vi "GetProperties.vi"(8 "error in":errorcluster, 11 "Path in":refnum<class "Path.lvclass">) -> (0 "error out":errorcluster, 3 "Path out":refnum<class "Path.lvclass">)   [LabVIEW 2014, in "Path.lvclass"]
uses:
  Path.lvclass
  Path.lvclass/Path.ctl
  Control/Control.lvclass
  Text/Text.lvclass
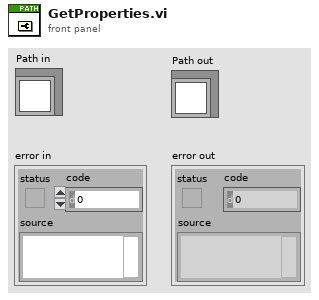
[diagram p1: front panel]
types:
  T1 = typedef "LVRectTypeDef.ctl" = cluster{"Left":i16, "Top":i16, "Right":i16, "Bottom":i16}
  T2 = typedef "LVBrowseOptionsTypeDef.ctl" = cluster{"Prompt":string, "Match Pattern":string, "select mode":enum32{"existing file", "new file", "new or existing file", "existing dir", "new dir", "new or existing dir", "existing file (use LLBs)", "new file (use LLBs)", "new or existing file (use LLBs)", "new or existing file or directory (use LLBs)", "existing dir (use LLBs)", "new dir (use LLBs)", "new or existing dir (use LLBs)", "existing file or dir", "new file or dir", "new or existing file or dir", "existing file or dir (use LLBs)", "new file or dir (use LLBs)"}, "Start Path":path, "Pattern Label":string, "Button Text":string}
  T3 = typedef "LVBoundsTypeDef.ctl" = cluster{"Width":u32, "Height":u32}
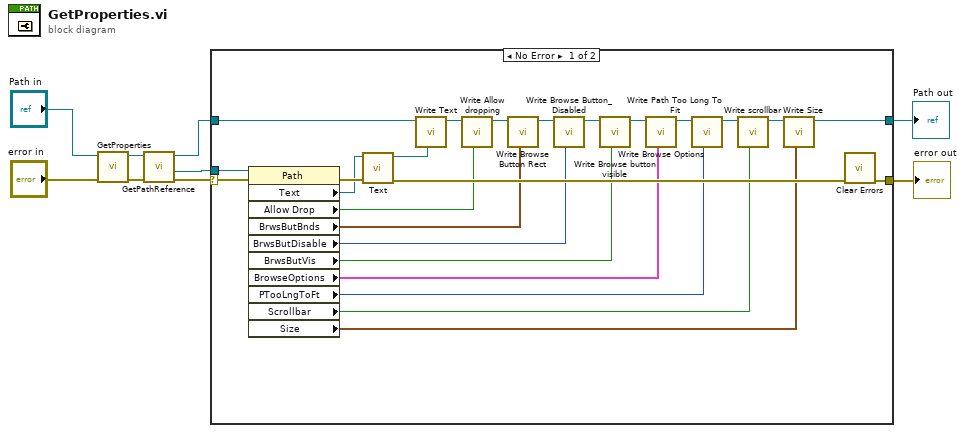
[diagram p0: block diagram]
diagram:
  n1 = call-parent "GetProperties.vi"("error in"="error in", "Control in"="Path in") -> ("error out"=w6:errorcluster, "Control out"=w7:refnum<class "Path.lvclass">)  [unwired: 8 in]
  n2 = call "GetPathReference.vi"("error in"=w6, "Path in"=w7) -> ("error out"=w4:errorcluster, "path reference"=w5:refnum<vi>, "Path out"=w3:refnum<class "Path.lvclass">)  [unwired: 7 in]
  n3 = case shown="No Error" w4 {
    selector: w4 -> [w33 w36]
    tunnel: w5 -> [w34 _]
    tunnel: w3 -> [w20 w35]
    tunnel: [w25 w35] -> w1
    tunnel: [w10 w36] -> w2
    frame No Error {
      n4 = property class="Path"(reference=w34, error in=w33) -> (error out=w23:errorcluster, "Text"=w22:refnum<vi>, "Allow Drop"=w18:bool, "BrwsButBnds"=w17:T1, "BrwsButDisable"=w16:u8, "BrwsButVis"=w15:bool, "BrowseOptions"=w14:T2, "PTooLngToFt"=w13:enum32{"Abbreviate Path", "Clip Path"}, "Scrollbar"=w12:bool, "Size"=w11:T3)  [unwired: 1 out]
      n5 = call "Text.vi"("error in"=w23, "GObj Refnum"=w22) -> ("error out"=w19:errorcluster, "Text out"=w21:refnum<class "Text.lvclass">)  [unwired: 8 in]
      n6 = call "Write Text.vi"("Text"=w21, "Path in"=w20) -> ("Path out"=w24:refnum<class "Path.lvclass">)  [unwired: 7 in]
      n7 = call "Write Allow dropping.vi"("Allow dropping"=w18, "Path in"=w24) -> ("Path out"=w32:refnum<class "Path.lvclass">)  [unwired: 7 in]
      n8 = call "Write Browse Button Rect.vi"("Browse Button Rect"=w17, "Path in"=w32) -> ("Path out"=w31:refnum<class "Path.lvclass">)  [unwired: 7 in]
      n9 = call "Write Browse Button_Disabled.vi"("Browse Button:Disabled"=w16, "Path in"=w31) -> ("Path out"=w30:refnum<class "Path.lvclass">)  [unwired: 7 in]
      n10 = call "Write Browse button visible.vi"("Browse button visible"=w15, "Path in"=w30) -> ("Path out"=w29:refnum<class "Path.lvclass">)  [unwired: 7 in]
      n11 = call "Write Browse Options.vi"("Browse Options"=w14, "Path in"=w29) -> ("Path out"=w28:refnum<class "Path.lvclass">)  [unwired: 7 in]
      n12 = call "Write Path Too Long To Fit.vi"("Path Too Long To Fit"=w13, "Path in"=w28) -> ("Path out"=w27:refnum<class "Path.lvclass">)  [unwired: 7 in]
      n13 = call "Write scrollbar.vi"("scrollbar"=w12, "Path in"=w27) -> ("Path out"=w26:refnum<class "Path.lvclass">)  [unwired: 7 in]
      n14 = call "Write Size.vi"("Size"=w11, "Path in"=w26) -> ("Path out"=w25:refnum<class "Path.lvclass">)  [unwired: 7 in]
      n15 = call <vilib>:"Clear Errors.vi"("error in (no error)"=w19) -> ("error out"=w10:errorcluster)  [unwired: 5 in, 1 out]
    }
    frame Error {
    }
  }
  "error out" <- w2
  "Path out" <- w1
